vi "Aktualizacja listy z punktami do usunięcia.vi"(9 "index column name add":i32, 10 "Lista współrzędnych":string[][](array[string]), 11 "Lista z punktami do usunięcia":refnum<vi>) -> ()   [LabVIEW 2015, in "Biblioteka moduł map v3.lvlib" / "Obsługa listy współrzędnych.lvlib"]
doc: "Dodanie do kontrolki enumerate nazw wszystkich punktów znajdujących sie na liście współrzędnych."
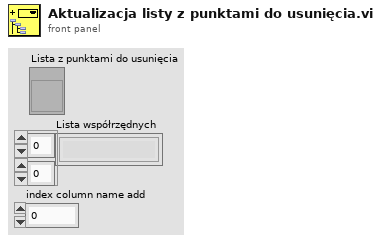
[diagram p1: front panel]
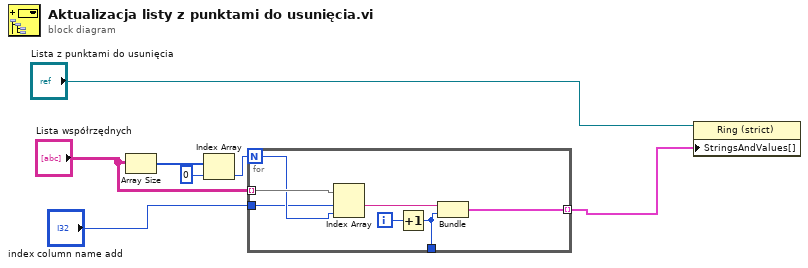
[diagram p0: block diagram]
diagram:
  n1 = Array Size(array="Lista współrzędnych") -> (size(s)=w5:i32[])
  n2 = Index Array(array=w5, index=0) -> (element=w3:i32)
  n3 = for {
    N: w3 -> [w10]
    tunnel: "Lista współrzędnych" -> [w14] mode=indexing
    tunnel: [w12] -> w2 mode=indexing
    tunnel: [w9] -> _
    tunnel: "index column name add" -> [w8]
    i -> [w11]
    n4 = Index Array(array=w14, index #1=w8, index #2=w10) -> (element #1=w13:string)  [unwired: 1 out]
    n5 = Increment(x=w11) -> (x+1=w9:i32)
    n6 = Bundle(w13, w9) -> (w12:cluster{string, i32})  [unwired: 1 in]
  }
  n7 = property class="Ring (strict)"(reference="Lista z punktami do usunięcia", "StringsAndValues[]"=w2) -> ()  [unwired: 1 in, 2 out]
